vi "PyLoN_SRS1.vi"() -> ()   [LabVIEW 2014]
uses:
  C:/Users/wrsilva/Desktop/Labview VIs/PIXIS_TEST/SITK_Labview/Examples70_2_2_0_1/RS Pixis/MaxY.vi
  C:/Users/wrsilva/Desktop/Labview VIs/PIXIS_TEST/SITK_Labview/Examples70_2_2_0_1/RS Pixis/MaxX.vi
  <vilib>/Utility/file.llb/Write To Spreadsheet File (DBL).vi
panel:
  in  "?":bool
  in  "?":T1(tab)
  in  "Shutter State":u16(ring)=2 items=["Always Close", "Open Each Exposure", "Open Until Finish", "Open waiting for triger"]
  in  "Trigger Edge":u16(ring) items=["Positive", "Negative"]
  in  "Timing Mode":u16(ring) items=["Free Run", "Triger First", "Ext Sync", "Bulb Mode", "Variable Mode", "Flash Mode"]
  in  "ADC Speed":u16(ring)=2 items=["ADC Slow", "ADC Fast", "Default"]
  in  "ADC Gain":u16(ring) items=["ADC Low", "ADC High"]
  in  "Temperature":dbl=-100.0 caption="SET Temperature" format="%.2f"
  in  "Skip Serial  Reg Clean":dbl=1.0 format="%.2f"
  in  "Vertical Timing":dbl=3.2
  out "Vertical Timing":dbl
  in  "Readout Port":i32=4 min=-1 step=1
  in  "?":T2={"X start"=0, "X end"=1023, "X Binning/Grouping"=1, "Y start"=0, "Y end"=1, "Y Binning/Grouping"=1}
  in  "Logic Out":u16(ring) items=["Not Scan", "Shutter", "Not Rady", "Logic 0", "Clearing", "Not Ft Image Shift", "Reserved", "Logic1", "Expos Prog", "Expos", "Image Shift", "Readout", "Acquiring", "Wait For Trig"]
  in  "Use Custom Chip":bool
  in  "?":bool
  in  "Exposure Time (s)":dbl=0.004 min=0.0 step=0.001 format="%.3f"
  in  "?":bool
  in  "?":bool
  out "?":u16[](graph)
  in  "file path":path
  in  "File_name":string
  in  "# of spectrum per frame":i32
  in  "# of Frames":i32
  in  "FLIP SPECTRA":bool
  in  "?":bool
  in  "?":bool
  in  "?":bool
  out "?":dbl[](graph)
  in  "?":bool
  in  "Number of Images":u32=1 min=1 step=1
  out "?":dbl[](graph)
  in  "?":bool
  in  "# of Sets":i32
  out "Current Set":u32=24
  in  "#Ground per set":u32=3
  in  "Timepoints":dbl[](array[numeric])=[200.0, 100.0, 300.0, 400.0, 500.0]
  in  "File Path":path
  in  "File Name":string
  in  "Ground State\nSubstract?":bool
  in  "PyLonN Error In":errorcluster
  out "PyLoN Error Out":errorcluster
  out "PyLoN Ready":bool
  out "PyLoN \nTemperature":dbl
  # "REGION OF INTEREST"
  # "TRIGGER"
  # "ADC"
  # "SHUTTER"
  # "INPUT VARIABLES"
  # "TTL LOGIC"
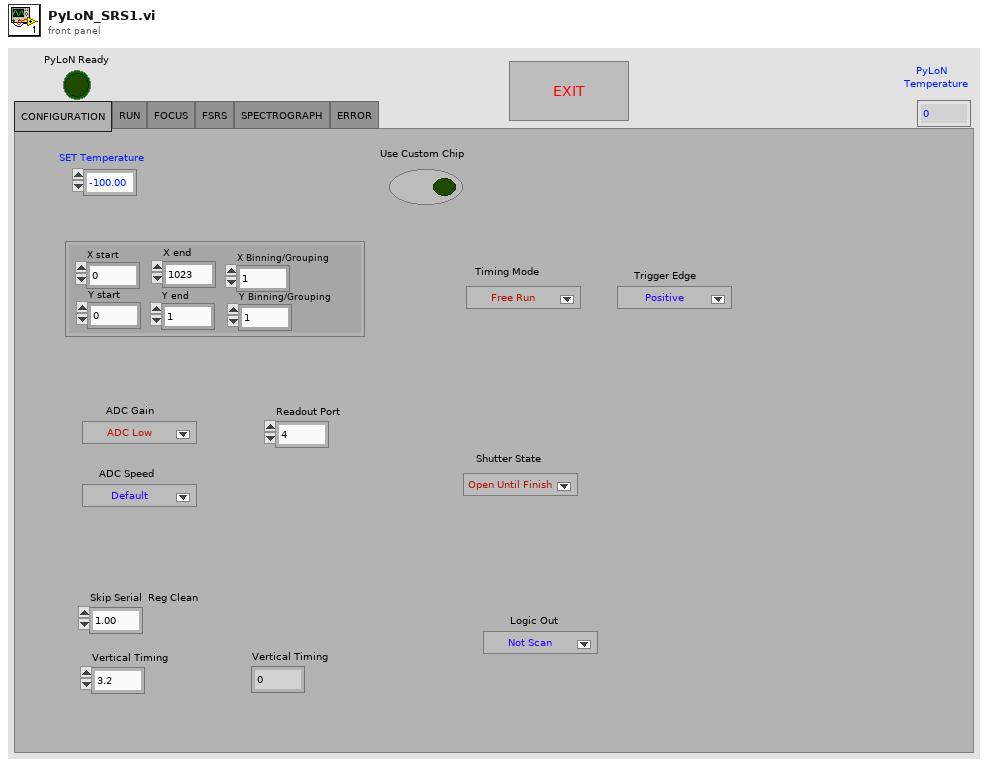
[diagram p1: front panel]
types:
  T1 = enum32{"CONFIGURATION", "RUN", "FOCUS", "FSRS", "SPECTROGRAPH", "ERROR"}
  T2 = cluster{"X start":u32, "X end":u32, "X Binning/Grouping":u32, "Y start":u32, "Y end":u32, "Y Binning/Grouping":u32}
  T3 = enum32{"Initializing", "RUN", "FSRS", "Monochromator", "Errors"}
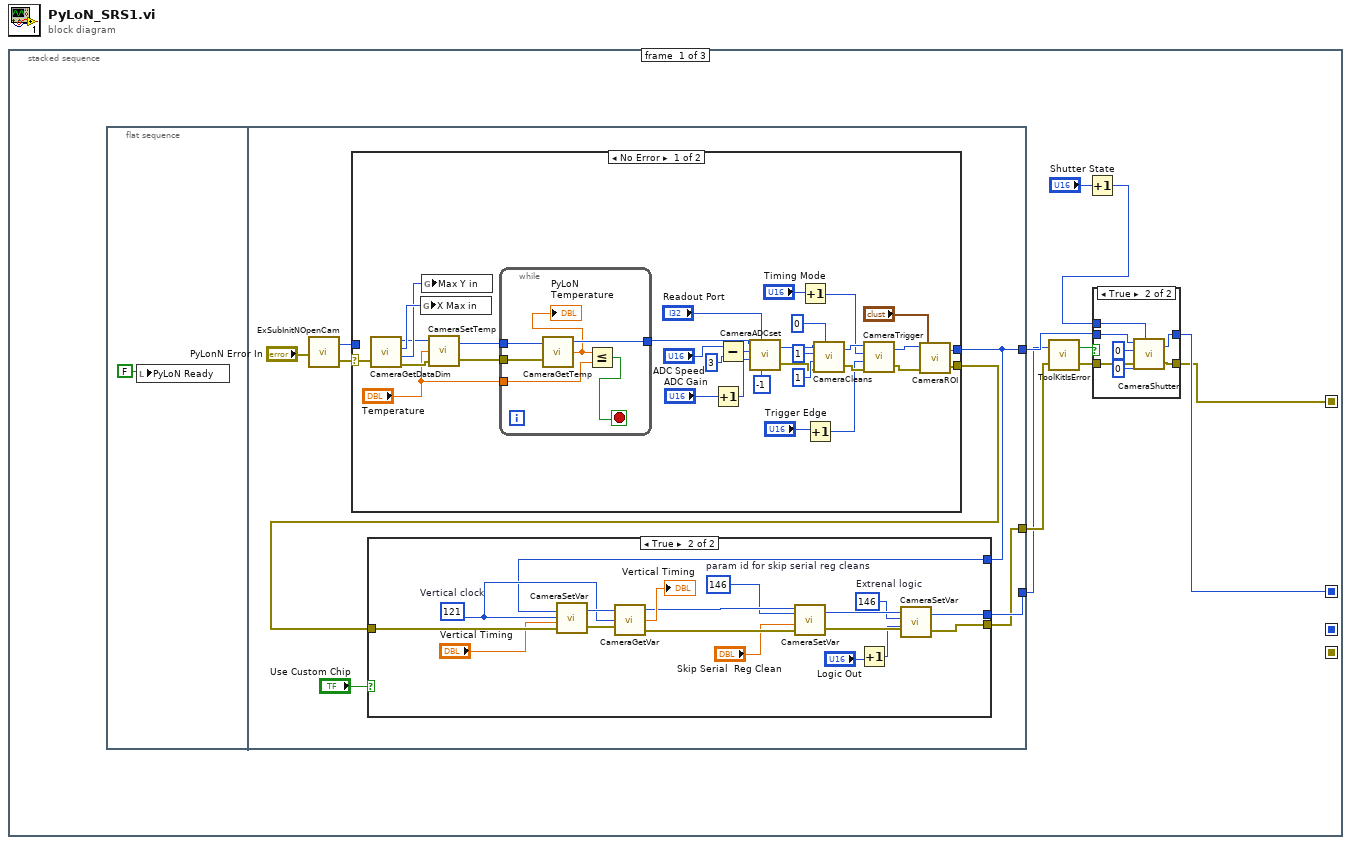
[diagram p0: block diagram]
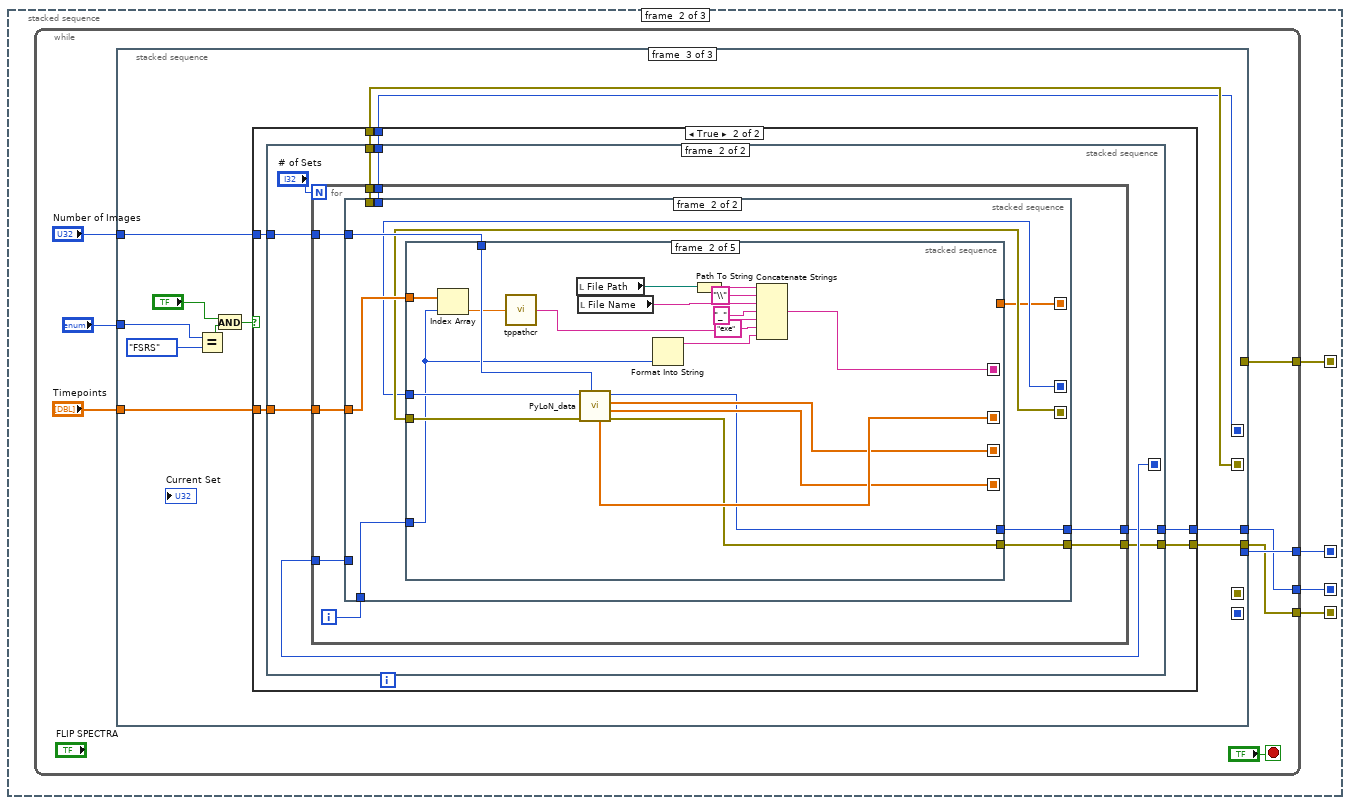
[diagram p5: hidden frame]
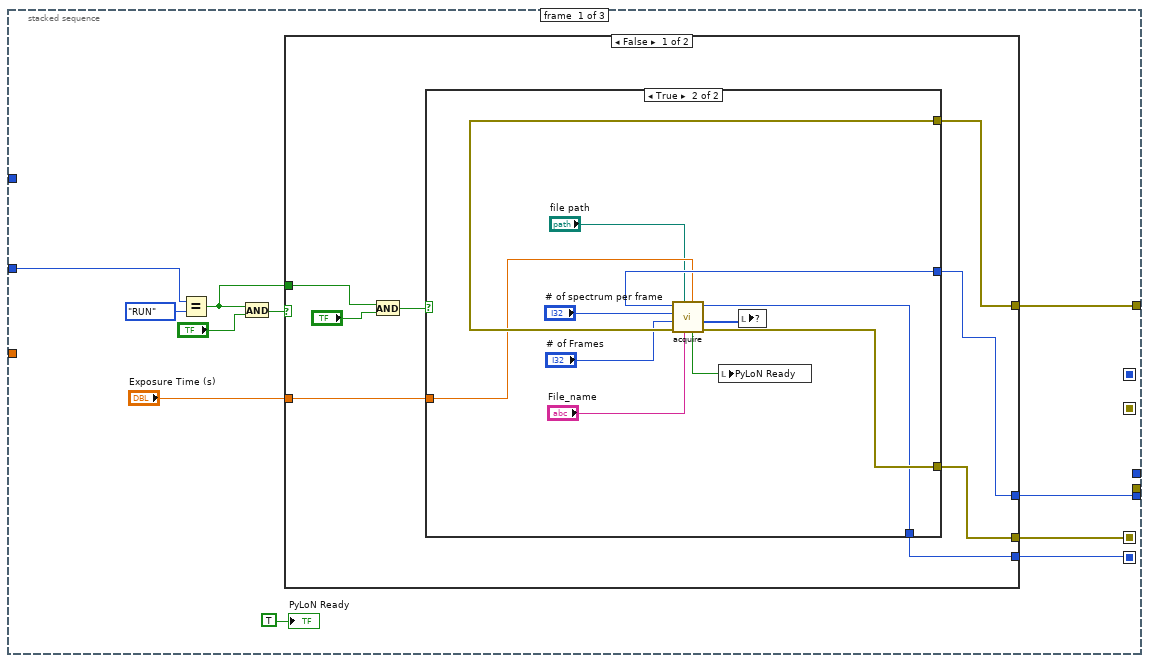
[diagram p6: hidden frame]
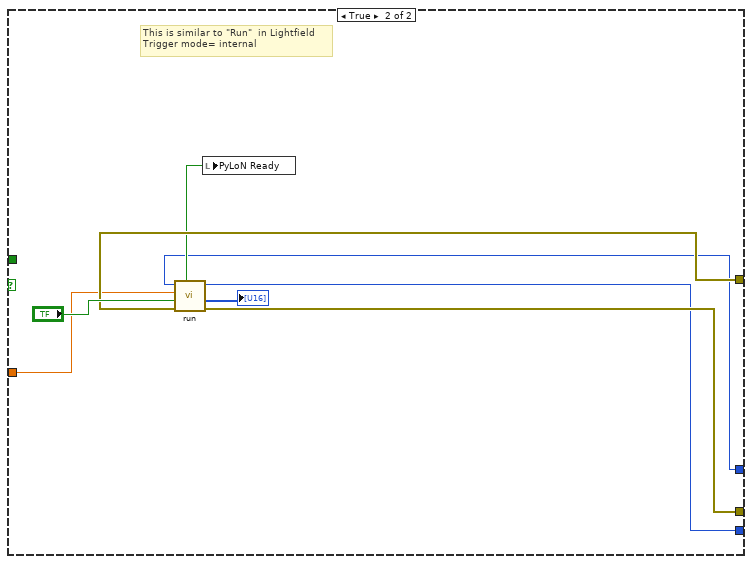
[diagram p8: hidden frame]
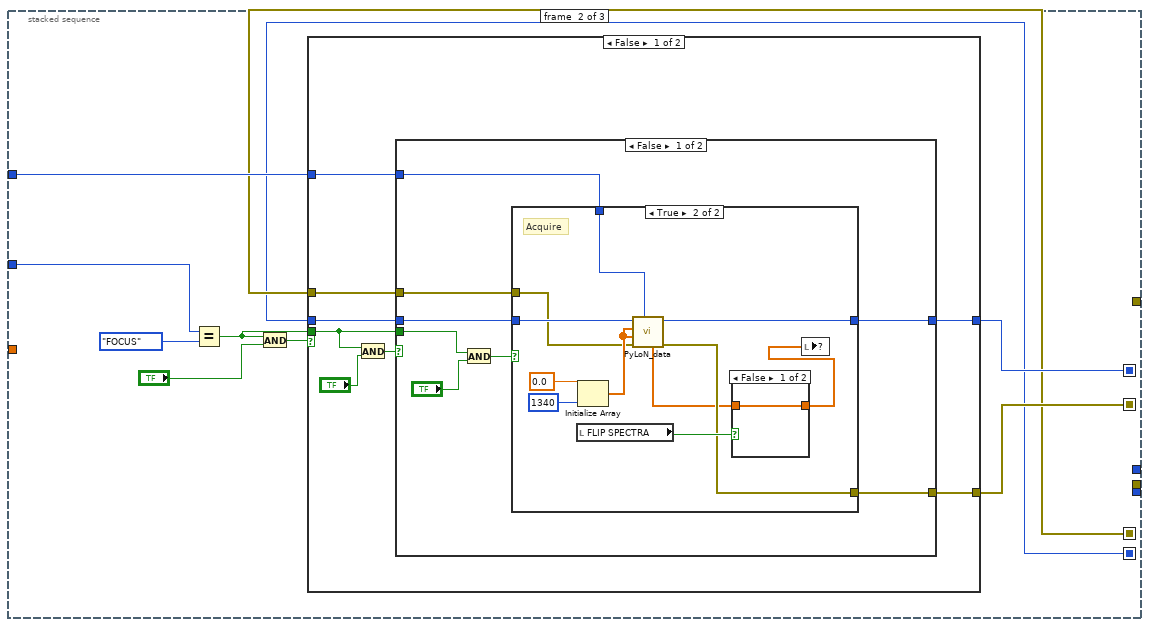
[diagram p9: hidden frame]
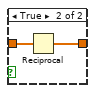
[diagram p11: hidden frame]
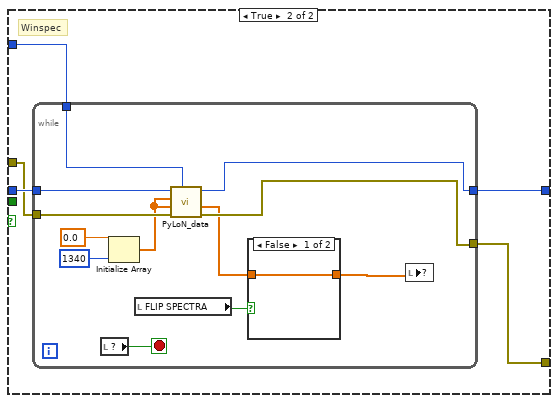
[diagram p12: hidden frame]
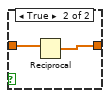
[diagram p13: hidden frame]
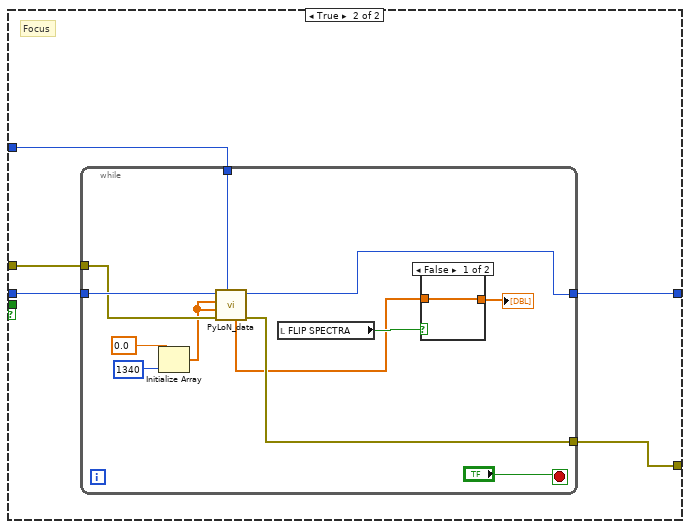
[diagram p14: hidden frame]
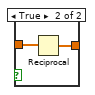
[diagram p15: hidden frame]
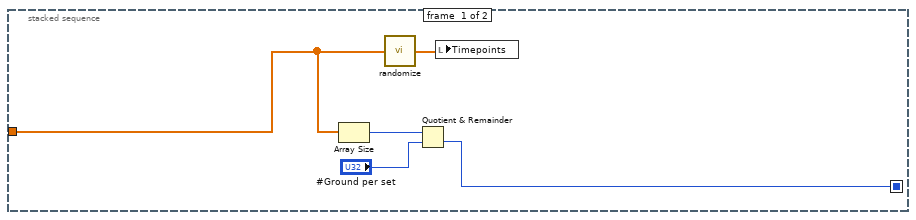
[diagram p17: hidden frame]
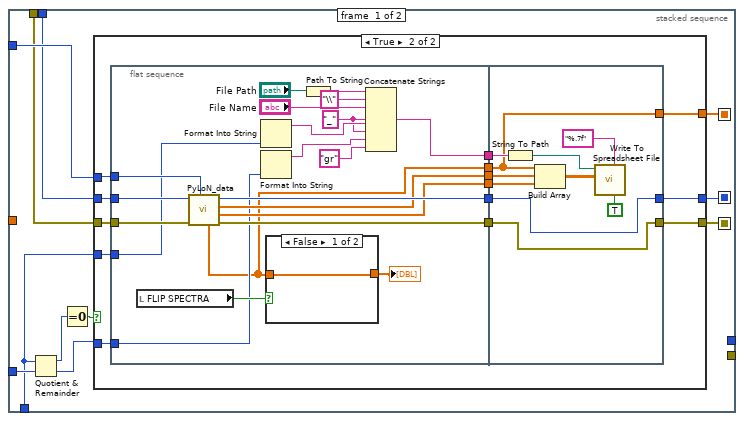
[diagram p18: hidden frame]
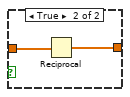
[diagram p20: hidden frame]
diagram:
  n1 = stacked-sequence {
    seq-local: [w4 _ _] -> [_ w90 _]
    seq-local: [w7 _ _] -> [_ w91 _]
    seq-local: [_ w89 _] -> [_ _ w381]
    seq-local: [_ w88 _] -> [_ _ w380]
    frame #0 {
      n2 = flat-sequence {
        tunnel: [w15] -> w9
        tunnel: [w12] -> w6
        tunnel: [w13] -> w3
        frame #0 {
          n3 = local write "PyLoN Ready"(FALSE ("PyLoN Ready")) -> ()
        }
        frame #1 {
          n4 = call "ExSubInitNOpenCam.vi"("error in (no error)"="PyLonN Error In") -> ("Camera Handle"=w16:u32, "error out"=w17:errorcluster)
          n5 = case shown="No Error" w17 {
            selector: w17 -> [w39 w78]
            tunnel: w16 -> [_ w77]
            tunnel: [w50 w77] -> w15
            tunnel: [w49 w78] -> w14
            frame No Error {
              n6 = call <userlib>:"CameraGetDataDim.vi"("error in"=w39) -> ("Camera Handle"=w68:u32, "Xdim"=w70:u32, "Ydim"=w69:u32, "error out"=w67:errorcluster)  [unwired: 1 in]
              n7 = global write "MaxX.vi" "X Max in"(w70) -> ()
              n8 = global write "MaxY.vi" "Max Y in"(w69) -> ()
              n9 = call <userlib>:"CameraSetTemp.vi"("error in (no error)"=w67, "Temperature"="Temperature", "Camera Handle"=w68) -> ("error out"=w53:errorcluster, "Camera Handle"=w54:u32)
              n10 = while {
                tunnel: w54 -> [w76]
                tunnel: w53 -> [w75]
                tunnel: "Temperature" -> [w74]
                tunnel: [w72] -> w51
                stop <- w73 stop-if-true
                n11 = call <userlib>:"CameraGetTemp.vi"("Camera Handle"=w76, "error in (no error)"=w75) -> ("Camera Handle"=w72:u32, "Temperature"=w71:dbl)  [unwired: 1 out]
                "PyLoN \nTemperature" <- w71
                n12 = Less Or Equal?(x=w71, y=w74) -> (x <= y?=w73:bool)
              }
              n13 = Increment(x="ADC Gain") -> (x+1=w65:u16)
              n14 = Subtract(x="ADC Speed", y=u16 3) -> (x-y=w47:u16)
              n15 = call <userlib>:"CameraADCset.vi"("ADC offset"=-1, "Read Out port"="Readout Port", "ADC Gain"=w65, "ADC Speed"=w47, "Camera Handle"=w51) -> ("error out"=w57:errorcluster, "Camera Handle"=w63:u32)  [unwired: 1 in]
              n16 = Increment(x="Timing Mode") -> (x+1=w42:u16)
              n17 = Increment(x="Trigger Edge") -> (x+1=w40:u16)
              n18 = call <userlib>:"CameraCleans.vi"("Camera Handle"=w63, "Number of Clears"=u32 1, "Number of Strips Per Clear"=u32 1, "error in"=w57, "Continuous Clears"=u32 0) -> ("Camera Handle"=w62:u32, "error out"=w56:errorcluster)
              n19 = call <userlib>:"CameraTrigger.vi"("error in"=w56, "Trigger Edge"=w40, "Timing Mode"=w42, "Camera Handle"=w62) -> ("error out"=w55:errorcluster, "Camera Handle"=w61:u32)
              n20 = call <userlib>:"CameraROI.vi"("error in"=w55, "ROI Params"="?", "Camera Handle"=w61) -> ("error out"=w49:errorcluster, "Camera Handle"=w50:u32)  [unwired: 1 in]
            }
            frame Error {
            }
          }
          n21 = case shown="True" "Use Custom Chip" {
            tunnel: w15 -> [w19 w34]
            tunnel: w14 -> [w20 w33]
            tunnel: [w19 w27] -> w13
            tunnel: [w20 w25] -> w12
            frame False {
            }
            frame True {
              w24 = 146  # Extrenal logic
              w29 = 146  # param id for skip serial reg cleans
              w37 = u32 121  # Vertical clock
              n22 = call <userlib>:"CameraSetVar.vi"("error in"=w33, "Value"="Vertical Timing", "Parameter ID"=w37, "Camera Handle"=w34) -> ("error out"=w36:errorcluster, "CameraHandle"=w38:u32)
              n23 = call <userlib>:"CameraGetVar.vi"("error in"=w36, "Parameter ID"=w37, "Camera Handle"=w38) -> ("error out"=w31:errorcluster, "Value"=→"Vertical Timing":dbl, "Camera Handle"=w32:u32)
              n24 = call <userlib>:"CameraSetVar.vi"("error in"=w31, "Value"="Skip Serial  Reg Clean", "Parameter ID"=w29, "Camera Handle"=w32) -> ("error out"=w26:errorcluster, "CameraHandle"=w28:u32)
              n25 = Increment(x="Logic Out") -> (x+1=w22:u16)
              n26 = call <userlib>:"CameraSetVar.vi"("error in"=w26, "Value"=w22, "Parameter ID"=w24, "Camera Handle"=w28) -> ("error out"=w25:errorcluster, "CameraHandle"=w27:u32)
            }
          }
        }
      }
      n27 = call <userlib>:"ToolKitIsError.vi"("error in"=w6, "Reserved"=w3) -> ("error out"=w5:errorcluster, "Error Flag"=w8:bool)
      n28 = Increment(x="Shutter State") -> (x+1=w1:u16)
      n29 = case shown="True" w8 {
        tunnel: w9 -> [w80 w85]
        tunnel: [w79 w84] -> w4
        tunnel: [w80 w83] -> w7
        tunnel: w5 -> [w79 w82]
        tunnel: w1 -> [_ w81]
        frame False {
        }
        frame True {
          n30 = call <userlib>:"CameraShutter.vi"("Camera Handle"=w85, "Shutter Comp Time: Pre Open"=u32 0, "Shutter Comp Time: Post Open"=u32 0, "error in"=w82, "Shutter State"=w81) -> ("Camera Handle"=w83:u32, "error out"=w84:errorcluster)
        }
      }
    }
    frame #1 {
      n31 = while {
        tunnel: w91 -> [w99]
        tunnel: w90 -> [w98]
        tunnel: [w93] -> w89
        tunnel: [w92] -> w88
        stop <- "?" stop-if-true
        n32 = stacked-sequence {
          seq-local: [_ w144 _] -> [_ _ w226]
          seq-local: [_ w143 _] -> [_ _ w228]
          seq-local: [w103 _ _] -> [_ w141 _]
          seq-local: [w104 _ _] -> [_ w142 _]
          tunnel: w99 -> [w101 _ _]
          tunnel: w98 -> [w110 _ _]
          tunnel: "?" -> [w105 w149 w232]
          tunnel: "Number of Images" -> [_ w147 w229]
          tunnel: "Timepoints" -> [_ _ w225]
          tunnel: [_ _ w224] -> w93
          tunnel: [_ _ w223] -> w92
          frame #0 {
            n33 = Equal?(x=w105, y=T3."RUN") -> (x = y?=w102:bool)
            n34 = And(x=w102, y="?") -> (x .and. y?=w107:bool)
            n35 = case shown="False" w107 {
              tunnel: w110 -> [w115 w135]
              tunnel: [w112 w137] -> w103
              tunnel: [w114 w138] -> w104
              tunnel: w102 -> [w118 _]
              tunnel: w101 -> [w113 w133]
              tunnel: "Exposure Time (s)" -> [w111 w132]
              frame False {
                n36 = And(x=w118, y="?") -> (x .and. y?=w116:bool)
                n37 = case shown="True" w116 {
                  tunnel: w115 -> [w120 w131]
                  tunnel: [w120 w130] -> w114
                  tunnel: w113 -> [w119 w129]
                  tunnel: [w119 w128] -> w112
                  tunnel: w111 -> [_ w125]
                  frame False {
                  }
                  frame True {
                    n38 = call "acquire.vi"("Exposure Time (s)"=w125, "File_name"="File_name", "file path"="file path", "error in (no error)"=w131, "# of Frames"="# of Frames", "# of spectrum per frame"="# of spectrum per frame", "Camera Handle"=w129) -> ("error out"=w130:errorcluster, 1:w121:u16[], "Camera Handle"=w128:u32, "PyLoN Ready"=w122:bool)  [unwired: 1 in]
                    n39 = local write "PyLoN Ready"(w122) -> ()
                    n40 = local write item#9(w121) -> ()
                  }
                }
              }
              frame True {
                # "This is similar to \"Run\"  in Lightfield\nTrigger mode= internal"
                n41 = call "run.vi"("error in (no error)"=w135, 9:"?", "Exposure Time (s)"=w132, "Camera Handle"=w133) -> ("error out"=w138:errorcluster, 1:→"?":u16[], "Camera Handle 2"=w137:u32, "PyLoN Ready"=w134:bool)  [unwired: 4 in]
                n42 = local write "PyLoN Ready"(w134) -> ()
              }
            }
            "PyLoN Ready" <- TRUE
          }
          frame #1 {
            n43 = Equal?(x=w149, y=T1."FOCUS") -> (x = y?=w145:bool)
            n44 = And(x=w145, y="?") -> (x .and. y?=w148:bool)
            n45 = case shown="False" w148 {
              tunnel: w141 -> [w157 w206]
              tunnel: [w153 w205] -> w144
              tunnel: w142 -> [w155 w204]
              tunnel: w147 -> [w156 w203]
              tunnel: [w154 w202] -> w143
              tunnel: w145 -> [w150 _]
              frame False {
                n46 = And(x=w150, y="?") -> (x .and. y?=w152:bool)
                n47 = case shown="False" w152 {
                  tunnel: w157 -> [w160 w186]
                  tunnel: w156 -> [w161 w185]
                  tunnel: w155 -> [w162 w184]
                  tunnel: [w158 w183] -> w154
                  tunnel: [w159 w182] -> w153
                  tunnel: w150 -> [w163 _]
                  frame False {
                    n48 = And(x=w163, y="?") -> (x .and. y?=w165:bool)
                    n49 = case shown="True" w165 {
                      tunnel: w162 -> [w166 w171]
                      tunnel: w161 -> [_ w174]
                      tunnel: w160 -> [w167 w173]
                      tunnel: [w167 w169] -> w159
                      tunnel: [w166 w170] -> w158
                      frame False {
                      }
                      frame True {
                        # "Acquire"
                        n50 = local read "FLIP SPECTRA"() -> (w176:bool)
                        n51 = Initialize Array(0.0, u32 1340) -> (w172:dbl[])
                        n52 = call "PyLoN_data.vi"("Number of Images"=w174, "error in (no error)"=w171, "PumpOffBkgd"=w172, "PumpOnBkgd"=w172, "Camera Handle"=w173) -> ("error out"=w170:errorcluster, "Camera Handle 2"=w169:u32, "Raman_Gain"=w168:dbl[])  [unwired: 2 in, 2 out]
                        n53 = case shown="False" w176 {
                          tunnel: w168 -> [w179 w181]
                          tunnel: [w179 w180] -> w175
                          frame False {
                          }
                          frame True {
                            n54 = Reciprocal(x=w181) -> (1/x=w180:dbl[])
                          }
                        }
                        n55 = local write item#21(w175) -> ()
                      }
                    }
                  }
                  frame True {
                    # "Winspec"
                    n56 = while {
                      tunnel: w186 -> [w192]
                      tunnel: w185 -> [w193]
                      tunnel: [w187] -> w182
                      tunnel: w184 -> [w191]
                      tunnel: [w190] -> w183
                      stop <- w196 stop-if-true
                      n57 = local read item#27() -> (w196:bool)
                      n58 = Initialize Array(0.0, u32 1340) -> (w188:dbl[])
                      n59 = local read "FLIP SPECTRA"() -> (w195:bool)
                      n60 = call "PyLoN_data.vi"("Number of Images"=w193, "error in (no error)"=w191, "PumpOffBkgd"=w188, "PumpOnBkgd"=w188, "Camera Handle"=w192) -> ("error out"=w190:errorcluster, "Pump_Off"=w189:dbl[], "Camera Handle 2"=w187:u32)  [unwired: 2 in, 2 out]
                      n61 = case shown="False" w195 {
                        tunnel: w189 -> [w199 w200]
                        tunnel: [w199 w201] -> w194
                        frame False {
                        }
                        frame True {
                          n62 = Reciprocal(x=w200) -> (1/x=w201:dbl[])
                        }
                      }
                      n63 = local write item#21(w194) -> ()
                    }
                  }
                }
              }
              frame True {
                # "Focus"
                n64 = while {
                  tunnel: w204 -> [w211]
                  tunnel: w203 -> [w212]
                  tunnel: [w210] -> w202
                  tunnel: w206 -> [w213]
                  tunnel: [w208] -> w205
                  stop <- "?" stop-if-true
                  n65 = Initialize Array(0.0, u32 1340) -> (w209:dbl[])
                  n66 = call "PyLoN_data.vi"("Number of Images"=w212, "error in (no error)"=w211, "PumpOffBkgd"=w209, "PumpOnBkgd"=w209, "Camera Handle"=w213) -> ("error out"=w210:errorcluster, "Camera Handle 2"=w208:u32, "Raman_Gain"=w207:dbl[])  [unwired: 2 in, 2 out]
                  n67 = local read "FLIP SPECTRA"() -> (w215:bool)
                  n68 = case shown="False" w215 {
                    tunnel: w207 -> [w219 w221]
                    tunnel: [w219 w220] -> w214
                    frame False {
                    }
                    frame True {
                      n69 = Reciprocal(x=w221) -> (1/x=w220:dbl[])
                    }
                  }
                  "?" <- w214
                }
              }
            }
          }
          frame #2 {
            n70 = Equal?(x=w232, y=T1."FSRS") -> (x = y?=w230:bool)
            n71 = And(x="?", y=w230) -> (x .and. y?=w231:bool)
            n72 = case shown="True" w231 {
              tunnel: w229 -> [_ w240]
              tunnel: w226 -> [w233 w239]
              tunnel: w228 -> [w234 w238]
              tunnel: w225 -> [_ w237]
              tunnel: [w233 w236] -> w224
              tunnel: [w234 w235] -> w223
              frame False {
              }
              frame True {
                n73 = stacked-sequence {
                  seq-local: [w243 _] -> [_ w252]
                  tunnel: w240 -> [_ w251]
                  tunnel: w239 -> [_ w250]
                  tunnel: w238 -> [_ w249]
                  tunnel: w237 -> [w241 w248]
                  tunnel: [_ w247] -> w235
                  tunnel: [_ w246] -> w236
                  frame #0 {
                    n74 = Array Size(array=w241) -> (size(s)=w245:i32)
                    n75 = call "randomize.vi"("Input array"=w241) -> ("Output array"=w242:dbl[])
                    n76 = Quotient & Remainder(x=w245, y="#Ground per set") -> (floor(x/y)=w243:u32)  [unwired: 1 out]
                    n77 = local write "Timepoints"(w242) -> ()
                  }
                  frame #1 {
                    n78 = for {
                      N: "# of Sets" -> [_]
                      tunnel: w252 -> [w260]
                      tunnel: w251 -> [w259]
                      tunnel: w250 -> [w258]
                      tunnel: w249 -> [w257]
                      tunnel: w248 -> [w256]
                      tunnel: [w255] -> w247
                      tunnel: [w254] -> w246
                      i -> [w261]
                      n79 = stacked-sequence {
                        seq-local: [w263 _] -> [_ w326]
                        seq-local: [w264 _] -> [_ w327]
                        seq-local: [w262 _] -> [_ w325]
                        tunnel: w261 -> [w265 w328]
                        tunnel: w260 -> [w270 _]
                        tunnel: w259 -> [w268 w330]
                        tunnel: w258 -> [w267 _]
                        tunnel: w257 -> [w266 _]
                        tunnel: w256 -> [_ w329]
                        tunnel: [_ w324] -> w255
                        tunnel: [_ w323] -> w254
                        frame #0 {
                          n80 = Quotient & Remainder(x=w265, y=w270) -> (x-y*floor(x/y)=w271:u32, floor(x/y)=w269:u32)
                          n81 = Equal To 0?(x=w271) -> (x = 0?=w272:bool)
                          n82 = case shown="True" w272 {
                            tunnel: w269 -> [_ w284]
                            tunnel: w268 -> [_ w288]
                            tunnel: w267 -> [w274 w287]
                            tunnel: w266 -> [w273 w286]
                            tunnel: [w274 w277] -> w263
                            tunnel: [w273 w276] -> w264
                            tunnel: w265 -> [_ w285]
                            tunnel: [_ w275] -> w262
                            frame False {
                            }
                            frame True {
                              n83 = flat-sequence {
                                tunnel: w288 -> [w309]
                                tunnel: w287 -> [w308]
                                tunnel: w286 -> [w307]
                                tunnel: w285 -> [w295]
                                tunnel: w284 -> [w293]
                                tunnel: [w306] -> w283
                                tunnel: [w305] -> w282
                                tunnel: [w302] -> w281
                                tunnel: [w301] -> w280
                                tunnel: [w290] -> w279
                                tunnel: [w289] -> w278
                                tunnel: w283 -> [w315]
                                tunnel: w282 -> [w314]
                                tunnel: w281 -> [w318]
                                tunnel: w280 -> [w317]
                                tunnel: w279 -> [w319]
                                tunnel: w278 -> [w313]
                                tunnel: [w315] -> w277
                                tunnel: [w314] -> w276
                                tunnel: [w313] -> w275
                                frame #0 {
                                w294 = "_" ("string")
                                n84 = local read "FLIP SPECTRA"() -> (w304:bool)
                                n85 = call "PyLoN_data.vi"("Number of Images"=w309, "error in (no error)"=w307, "Camera Handle"=w308) -> ("error out"=w305:errorcluster, "Pump_Off"=w301:dbl[], "Pump_On"=w302:dbl[], "Camera Handle 2"=w306:u32, "Raman_Gain"=w289:dbl[])  [unwired: 4 in]
                                n86 = Format Into String(w295) -> (resulting string=w296:string)  [unwired: 3 in, 1 out]
                                n87 = Format Into String(w293) -> (resulting string=w292:string)  [unwired: 3 in, 1 out]
                                n88 = case shown="False" w304 {
                                tunnel: w289 -> [w310 w312]
                                tunnel: [w310 w311] -> w303
                                frame False {
                                }
                                frame True {
                                n89 = Reciprocal(x=w312) -> (1/x=w311:dbl[])
                                }
                                }
                                "?" <- w303
                                n90 = Path To String(path="File Path") -> (string=w300:string)
                                n91 = Concatenate Strings(w300, "\\" ("string"), "File Name", w294, w296, w294, w292, "gr" ("string")) -> (w290:string)
                                }
                                frame #1 {
                                n92 = String To Path(string=w319) -> (path=w320:path)
                                n93 = Build Array(w313, w318, w317) -> (w316:dbl[][])
                                n94 = call-poly <vilib>:"Write To Spreadsheet File.vi"("transpose? (no:F)"=TRUE, "format (%.3f)"="%.7f", "2D data"=w316, "file path (dialog if empty)"=w320) -> ()  [unwired: 4 in, 1 out]
                                }
                              }
                            }
                          }
                        }
                        frame #1 {
                          n95 = stacked-sequence {
                            seq-local: [_ w333 _ _ _] -> [_ _ _ w354 _]
                            seq-local: [_ w336 _ _ _] -> [_ _ _ w353 w360]
                            seq-local: [_ w335 _ _ _] -> [_ _ _ w352 _]
                            seq-local: [_ w334 _ _ _] -> [_ _ _ w351 _]
                            tunnel: w327 -> [_ w346 _ _ _]
                            tunnel: w326 -> [_ w345 _ _ _]
                            tunnel: w330 -> [_ w344 _ _ _]
                            tunnel: w329 -> [_ w341 _ _ _]
                            tunnel: w328 -> [_ w337 _ _ _]
                            tunnel: w325 -> [_ _ _ _ w361]
                            tunnel: [_ w332 _ _ _] -> w324
                            tunnel: [_ w331 _ _ _] -> w323
                            frame #0 {
                            }
                            frame #1 {
                              n96 = Index Array(array=w341, index=w337) -> (element=w340:dbl)
                              n97 = call "tppathcr.vi"("input"=w340) -> ("out"=w339:string)
                              n98 = local read "File Path"() -> (w343:path)
                              n99 = local read "File Name"() -> (w342:string)
                              n100 = call "PyLoN_data.vi"("Number of Images"=w344, "error in (no error)"=w346, "Camera Handle"=w345) -> ("error out"=w332:errorcluster, "Pump_Off"=w334:dbl[], "Pump_On"=w335:dbl[], "Camera Handle 2"=w331:u32, "Raman_Gain"=w336:dbl[])  [unwired: 4 in]
                              n101 = Format Into String(w337) -> (resulting string=w347:string)  [unwired: 3 in, 1 out]
                              n102 = Path To String(path=w343) -> (string=w350:string)
                              n103 = Concatenate Strings(w350, "\\" ("string"), w342, "_" ("string"), w339, "exe" ("string"), w347) -> (w333:string)
                            }
                            frame #2 {
                            }
                            frame #3 {
                              n104 = String To Path(string=w354) -> (path=w356:path)
                              n105 = Build Array(w353, w352, w351) -> (w355:dbl[][])
                              n106 = call-poly <vilib>:"Write To Spreadsheet File.vi"("transpose? (no:F)"=TRUE, "format (%.3f)"="%.7f", "2D data"=w355, "file path (dialog if empty)"=w356) -> ()  [unwired: 4 in, 1 out]
                            }
                            frame #4 {
                              n107 = case shown="False" "Ground State\nSubstract?" {
                                tunnel: w361 -> [_ w370]
                                tunnel: w360 -> [w364 w369]
                                frame False {
                                n108 = local read "FLIP SPECTRA"() -> (w363:bool)
                                n109 = case shown="True" w363 {
                                tunnel: [w365 w367] -> w362
                                tunnel: w364 -> [w365 w366]
                                frame False {
                                }
                                frame True {
                                n110 = Reciprocal(x=w366) -> (1/x=w367:dbl[])
                                }
                                }
                                n111 = local write item#33(w362) -> ()
                                }
                                frame True {
                                n112 = local read "FLIP SPECTRA"() -> (w371:bool)
                                n113 = case shown="False" w371 {
                                tunnel: [w374 w379] -> w373
                                tunnel: w370 -> [w375 w376]
                                tunnel: [w375 w378] -> w372
                                tunnel: w369 -> [w374 w377]
                                frame False {
                                }
                                frame True {
                                n114 = Reciprocal(x=w377) -> (1/x=w379:dbl[])
                                n115 = Reciprocal(x=w376) -> (1/x=w378:dbl[])
                                }
                                }
                                n116 = Subtract(x=w373, y=w372) -> (x-y=w368:dbl[])
                                n117 = local write item#33(w368) -> ()
                                }
                              }
                            }
                          }
                        }
                      }
                    }
                  }
                }
              }
            }
          }
        }
      }
    }
    frame #2 {
      n118 = local write "PyLoN Ready"(FALSE ("PyLoN Ready")) -> ()
      n119 = call "ExSubCloseCamUnInit.vi"("error in (no error)"=w380, "Camera Handle"=w381) -> ("error out"=→"PyLoN Error Out":errorcluster)
    }
  }
